vi "Flatten To String.vi"(8 "error in (no error)":errorcluster, 11 "iMessage in":refnum<class "iMessage.lvclass">) -> (0 "error out":errorcluster, 3 "data string":string)   [LabVIEW 2017, in "Message Interface.lvlib" / "iMessage.lvclass"]
uses:
  iMessage.lvclass
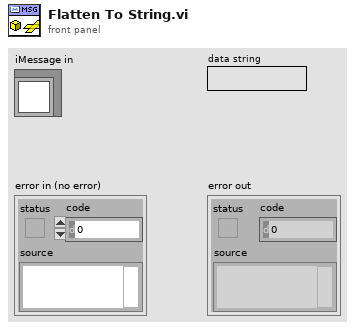
[diagram p1: front panel]
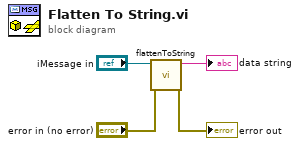
[diagram p0: block diagram]
diagram:
  n1 = call-dynamic "flattenToString.vi"("error in (no error)"="error in (no error)", "iMessage in"="iMessage in") -> ("error out"=→"error out":errorcluster, "data string"=→"data string":string)  [unwired: 8 in]
